vi "getMaxSpeed_DriveQuadTalonSRX.vi"() -> (1 "1 / Max Speed":dbl format="%.4f", 3 "Max Speed":dbl format="%.4f")   [LabVIEW 2019, in "DriveQuadTalonSRX_Motor.lvlib"]
uses:
  DriveQuadTalonSRX_Motor.lvlib
  globals_DriveQuadTalonSRX.vi
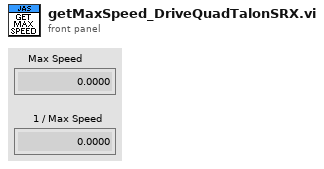
[diagram p1: front panel]
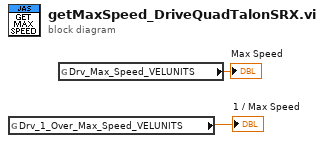
[diagram p0: block diagram]
diagram:
  n1 = global read "globals_DriveQuadTalonSRX.vi" "Drv_1_Over_Max_Speed_VELUNITS"() -> (→"1 / Max Speed":dbl)
  n2 = global read "globals_DriveQuadTalonSRX.vi" "Drv_Max_Speed_VELUNITS"() -> (→"Max Speed":dbl)
